vi "TransformObjectPosition.vi"(6 "Image time":dbl, 8 "error in (no error)":errorcluster, 9 "Pixel size":sgl, 10 "Objects":T2(array[cluster]) {"Aspect Ratio" format="%.2f"; "Orientation" format="%.2f"; "Area" format="%.2f"; "Object Center"."Y" format="%.2f"; "Object Center"."X" format="%.2f"}, 11 "Spacetime cluster":T1) -> (0 "error out":errorcluster, 1 "Focus out":dbl, 2 "Y out":dbl, 3 "X out":dbl)   [LabVIEW 2012]
panel:
  out "Y center":dbl(graph)
  out "X center":dbl(graph)
  out "X stage":dbl(graph)
  out "Y stage":dbl(graph)
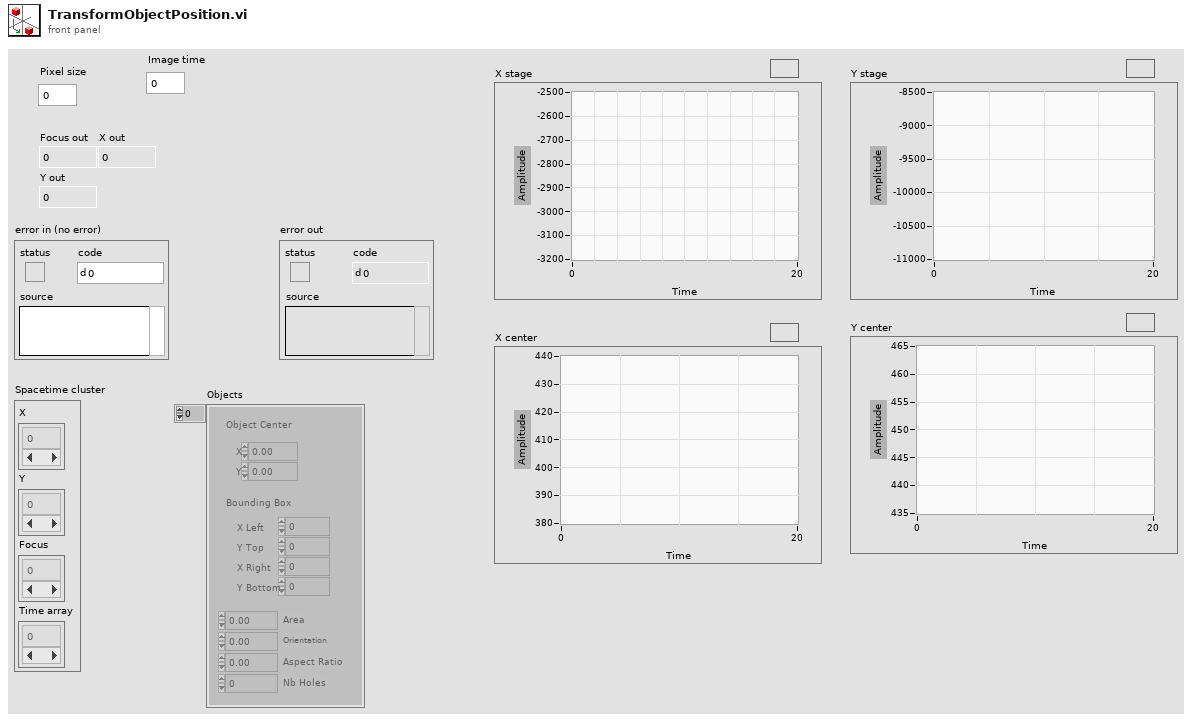
[diagram p1: front panel]
types:
  T1 = cluster{"X":dbl[], "Y":dbl[], "Focus":dbl[], "Time array":dbl[]}
  T2 = cluster{"Object Center":cluster{"X":sgl, "Y":sgl}, "Bounding Box":cluster{"X Left":i32, "Y Top":i32, "X Right":i32, "Y Bottom":i32}, "Area":sgl, "Orientation":sgl, "Aspect Ratio":sgl, "Nb Holes":i32}[]
  T3 = cluster{"Object Center":cluster{"X":sgl, "Y":sgl}, "Bounding Box":cluster{"X Left":i32, "Y Top":i32, "X Right":i32, "Y Bottom":i32}, "Area":sgl, "Orientation":sgl, "Aspect Ratio":sgl, "Nb Holes":i32}
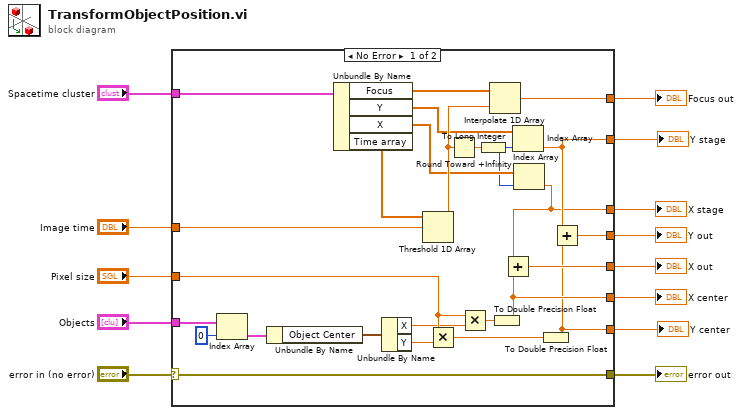
[diagram p0: block diagram]
diagram:
  n1 = case shown="No Error" "error in (no error)" {
    selector: "error in (no error)" -> [w26 w40]
    tunnel: [w26 w40] -> w12
    tunnel: "Objects" -> [w39 _]
    tunnel: "Pixel size" -> [w35 _]
    tunnel: "Image time" -> [w32 _]
    tunnel: [w29 _] -> w8
    tunnel: [w28 _] -> w7
    tunnel: [w27 _] -> w6
    tunnel: "Spacetime cluster" -> [w25 _]
    tunnel: [w17 _] -> w4
    tunnel: [w14 _] -> w3
    tunnel: [w22 _] -> w2
    tunnel: [w21 _] -> w1
    frame No Error {
      n2 = Index Array(array=w39, index=0) -> (element=w37:T3)
      n3 = Unbundle By Name(w37) -> ("Object Center"=w36:cluster{"X":sgl, "Y":sgl})
      n4 = Unbundle By Name(w25) -> ("Focus"=w24:dbl[], "Y"=w18:dbl[], "X"=w16:dbl[], "Time array"=w23:dbl[])
      n5 = Unbundle By Name(w36) -> ("X"=w34:sgl, "Y"=w33:sgl)
      n6 = Threshold 1D Array(2:w32, 3:w23) -> (0:w20:dbl)  [unwired: 1 in]
      n7 = Multiply(x=w35, y=w33) -> (x*y=w31:sgl)
      n8 = Round Toward +Infinity(x=w20) -> (ceil(x): smallest int >= x=w19:dbl)
      n9 = Multiply(x=w35, y=w34) -> (x*y=w30:sgl)
      n10 = To Long Integer(number=w19) -> (32bit integer=w15:i32)
      n11 = Interpolate 1D Array(1:w20, 2:w24) -> (0:w29:dbl)
      n12 = To Double Precision Float(number=w30) -> (double precision float=w22:dbl)
      n13 = Index Array(array=w18, index=w15) -> (element=w17:dbl)
      n14 = Index Array(array=w16, index=w15) -> (element=w14:dbl)
      n15 = Add(x=w14, y=w22) -> (x+y=w27:dbl)
      n16 = To Double Precision Float(number=w31) -> (double precision float=w21:dbl)
      n17 = Add(x=w17, y=w21) -> (x+y=w28:dbl)
    }
    frame Error {
    }
  }
  "error out" <- w12
  "Focus out" <- w8
  "Y out" <- w7
  "X out" <- w6
  "Y stage" <- w4
  "X stage" <- w3
  "X center" <- w2
  "Y center" <- w1
